vi "joystick_test.vi"() -> ()   [LabVIEW 2017]
uses:
  <vilib>/Utility/inputDevices.llb/joystickAcquire.vi
panel:
  in  "stop":bool
  out "direction info":T1
  out "button info":T2
  out "axis info":T3
  out "device ID":refnum<k1>
  out "joystick info":T4(array[cluster])
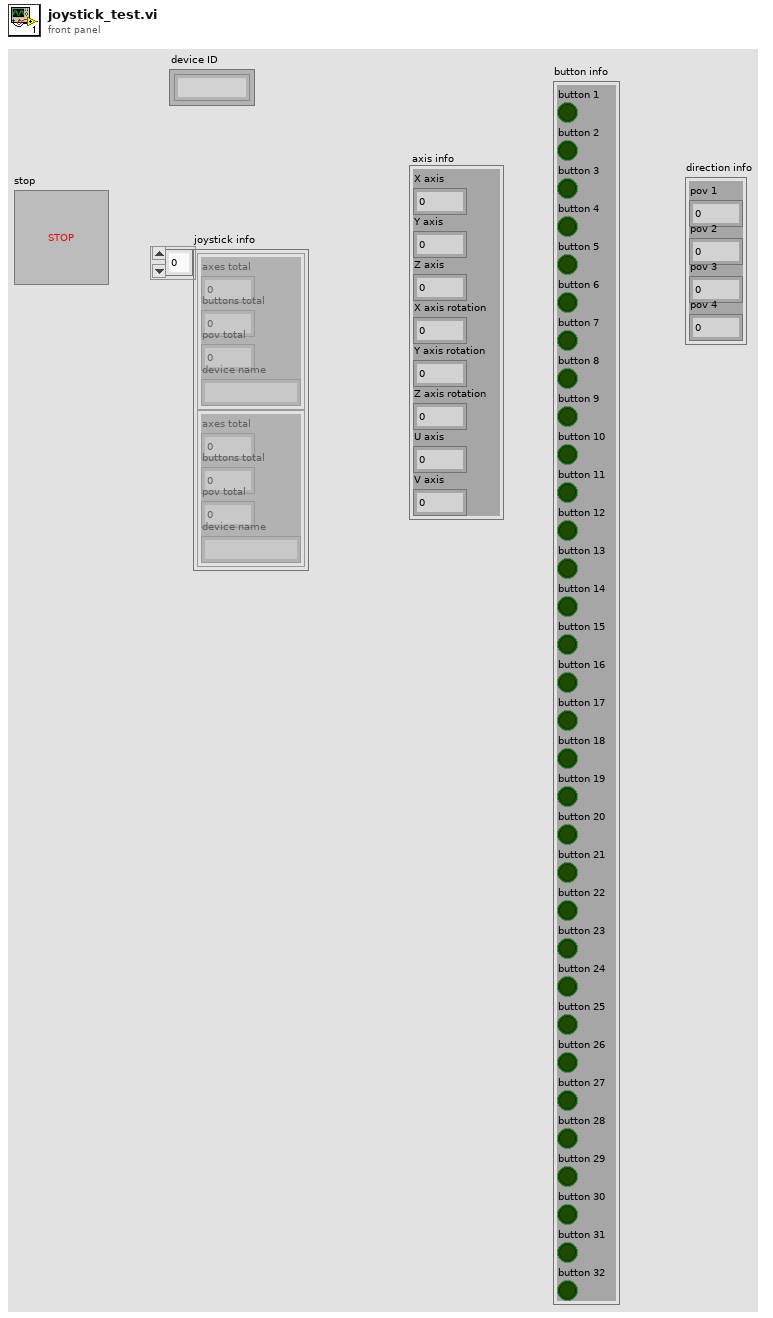
[diagram p1: front panel]
types:
  T1 = cluster{"pov 1":i32, "pov 2":i32, "pov 3":i32, "pov 4":i32}
  T2 = cluster{"button 1":bool, "button 2":bool, "button 3":bool, "button 4":bool, "button 5":bool, "button 6":bool, "button 7":bool, "button 8":bool, "button 9":bool, "button 10":bool, "button 11":bool, "button 12":bool, "button 13":bool, "button 14":bool, "button 15":bool, "button 16":bool, "button 17":bool, "button 18":bool, "button 19":bool, "button 20":bool, "button 21":bool, "button 22":bool, "button 23":bool, "button 24":bool, "button 25":bool, "button 26":bool, "button 27":bool, "button 28":bool, "button 29":bool, "button 30":bool, "button 31":bool, "button 32":bool}
  T3 = cluster{"X axis":i32, "Y axis":i32, "Z axis":i32, "X axis rotation":i32, "Y axis rotation":i32, "Z axis rotation":i32, "U axis":i32, "V axis":i32}
  T4 = cluster{"axes total":u32, "buttons total":u32, "pov total":u32, "device name":string}[]
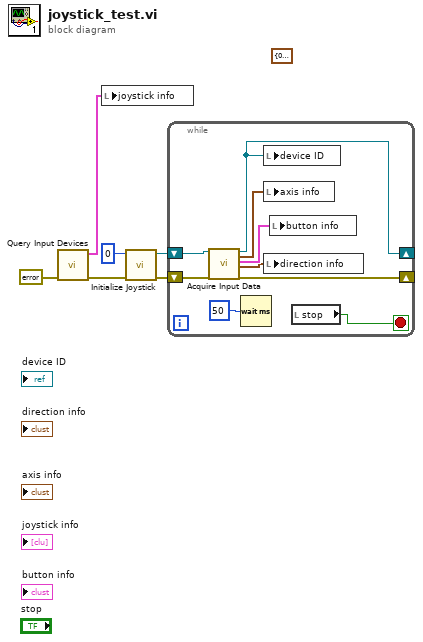
[diagram p0: block diagram]
diagram:
  (unwired) T3 {"X axis"=0, "Y axis"=-1, "Z axis"=0, "X axis rotation"=0, "Y axis rotation"=-1, "Z axis rotation"=0, "U axis"=0, "V axis"=0} ("axis info")
  n1 = call <vilib>:"Query Input Devices.vi"("error in (no error)"=errorcluster {"status"=FALSE, "code"=0, "source"=""}) -> ("error out"=w4:errorcluster, "joystick info"=w5:T4)  [unwired: 7 in, 2 out]
  n2 = local write "joystick info"(w5) -> ()
  n3 = call <vilib>:"Initialize Joystick.vi"("error in (no error)"=w4, "device index"=0) -> ("error out"=w1:errorcluster, "device ID"=w2:refnum<k1>)  [unwired: 8 in]
  n4 = while {
    shift-right: [w14] -> _
    shift-left: w1 -> [w12]
    shift-right: [w11] -> _
    shift-left: w2 -> [w13]
    stop <- w8 stop-if-true
    n5 = call-poly <vilib>:"Acquire Input Data.vi"("device ID"=w13, "error in (no error)"=w12) -> ("device ID"=w11:refnum<k1>, "axis info"=w7:T3, "button info"=w10:T2, "direction info"=w9:T1, "error out"=w14:errorcluster)  [unwired: 13 in]
    n6 = Wait (ms)(milliseconds to wait=u32 50) -> ()  [unwired: 1 out]
    n7 = local write "device ID"(w11) -> ()
    n8 = local write "axis info"(w7) -> ()
    n9 = local write "direction info"(w9) -> ()
    n10 = local write "button info"(w10) -> ()
    n11 = local read "stop"() -> (w8:bool)
  }
